vi "Update Enabled Items.vi"(10 "wheel type":string, 11 "enabled items in":T1={"Wheel Type"=TRUE, "X Position"=TRUE, "Y Position"=TRUE, "Frame Angle"=TRUE, "Wheel Name"=TRUE, "Wheel Radius"=TRUE, "Gear Ratio"=TRUE, "Forward Rotation Direction"=TRUE, "Steering Gear Ratio"=TRUE, "Motor Angle Offset"=TRUE, "Min Steering Angle"=TRUE, "Max Steering Angle"=TRUE, "Steering Range"=TRUE, "Caster Gear Ratio"=TRUE, "Forward Offset"=TRUE, "Roller Orientation"=TRUE}) -> (3 "enabled items out":T1={"Wheel Type"=TRUE, "X Position"=TRUE, "Y Position"=TRUE, "Frame Angle"=TRUE, "Wheel Name"=TRUE, "Wheel Radius"=TRUE, "Gear Ratio"=TRUE, "Forward Rotation Direction"=TRUE, "Steering Gear Ratio"=TRUE, "Motor Angle Offset"=TRUE, "Min Steering Angle"=TRUE, "Max Steering Angle"=TRUE, "Steering Range"=TRUE, "Caster Gear Ratio"=TRUE, "Forward Offset"=TRUE, "Roller Orientation"=TRUE})   [LabVIEW 2017, in "NI_Robotics_Configure Steering Frame.lvlib" / "User Defined Frame Subpanel.lvlib"]
uses:
  <vilib>/robotics/Dialog/Configure Steering Frame/User Defined Frame Subpanel/User Defined Frame Subpanel.lvlib
  <vilib>/robotics/Dialog/Configure Steering Frame/User Defined Frame Subpanel/Enabled Items.ctl
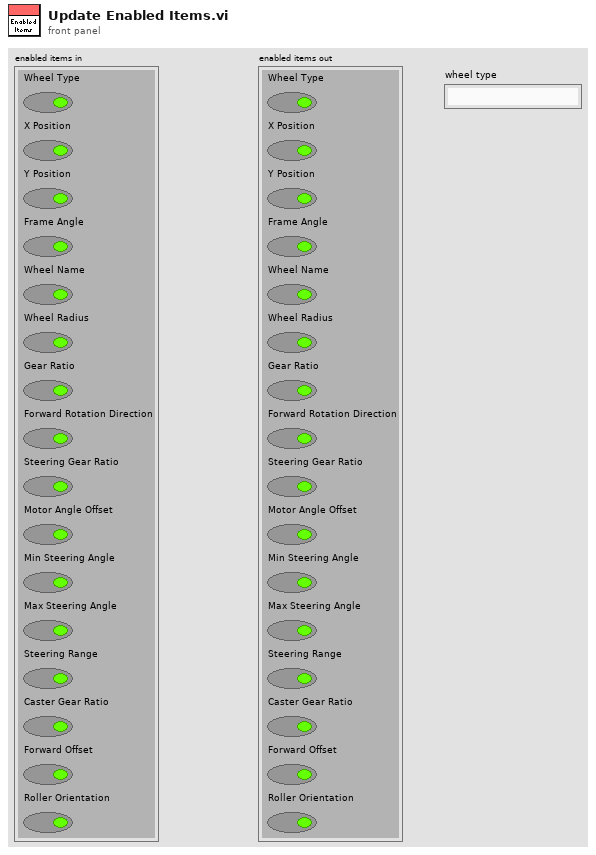
[diagram p1: front panel]
types:
  T1 = typedef "NI_Robotics_Configure Steering Frame.lvlib/User Defined Frame Subpanel.lvlib/Enabled Items.ctl" = cluster{"Wheel Type":bool, "X Position":bool, "Y Position":bool, "Frame Angle":bool, "Wheel Name":bool, "Wheel Radius":bool, "Gear Ratio":bool, "Forward Rotation Direction":bool, "Steering Gear Ratio":bool, "Motor Angle Offset":bool, "Min Steering Angle":bool, "Max Steering Angle":bool, "Steering Range":bool, "Caster Gear Ratio":bool, "Forward Offset":bool, "Roller Orientation":bool}
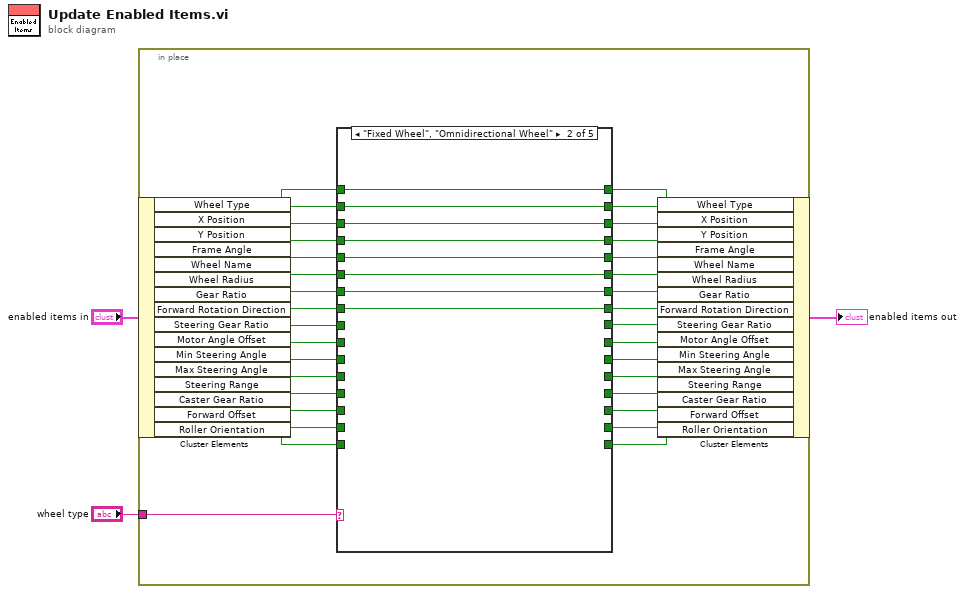
[diagram p0: block diagram]
diagram:
  n1 = in-place {
    in-place-border: "wheel type" -> [w36]
    n2 = in-place-cluster #1("enabled items in") -> ("Wheel Type"=w35:bool, "X Position"=w33:bool, "Y Position"=w31:bool, "Frame Angle"=w29:bool, "Wheel Name"=w27:bool, "Wheel Radius"=w25:bool, "Gear Ratio"=w23:bool, "Forward Rotation Direction"=w21:bool, "Steering Gear Ratio"=w19:bool, "Motor Angle Offset"=w17:bool, "Min Steering Angle"=w16:bool, "Max Steering Angle"=w15:bool, "Steering Range"=w14:bool, "Caster Gear Ratio"=w13:bool, "Forward Offset"=w12:bool, "Roller Orientation"=w11:bool)
    n3 = case shown="\"Fixed Wheel\", \"Omnidirectional Wheel\"" w36 {
      tunnel: w35 -> [w44 w52 w65 w75 w84]
      tunnel: [w44 w52 w65 w75 w84] -> w34
      tunnel: w33 -> [w43 w51 w64 w74 w83]
      tunnel: [w43 w51 w64 w74 w83] -> w32
      tunnel: w31 -> [w42 w50 w63 w73 w82]
      tunnel: [w42 w50 w63 w73 w82] -> w30
      tunnel: w29 -> [w41 w49 w62 w72 w81]
      tunnel: [w41 w49 w62 w72 w81] -> w28
      tunnel: w27 -> [w40 w48 w61 w71 w80]
      tunnel: [w40 w48 w61 w71 w80] -> w26
      tunnel: w25 -> [w39 w47 w60 w70 w79]
      tunnel: [w39 w47 w60 w70 w79] -> w24
      tunnel: w23 -> [w38 w46 w59 w69 w78]
      tunnel: [w38 w46 w59 w69 w78] -> w22
      tunnel: w21 -> [w37 w45 w57 w68 w77]
      tunnel: [w37 w45 w57 w68 w77] -> w20
      tunnel: w19 -> [_ _ w58 _ _]
      tunnel: [_ _ w58 _ _] -> w18
      tunnel: w17 -> [_ _ w56 _ _]
      tunnel: w16 -> [_ _ w55 _ _]
      tunnel: w15 -> [_ _ w54 _ _]
      tunnel: w14 -> [_ _ w53 _ _]
      tunnel: w13 -> [_ _ _ w67 _]
      tunnel: w12 -> [_ _ _ w66 _]
      tunnel: w11 -> [_ _ _ _ w76]
      tunnel: [_ _ w56 _ _] -> w10
      tunnel: [_ _ w55 _ _] -> w9
      tunnel: [_ _ w54 _ _] -> w8
      tunnel: [_ _ w53 _ _] -> w7
      tunnel: [_ _ _ w67 _] -> w6
      tunnel: [_ _ _ w66 _] -> w5
      tunnel: [_ _ _ _ w76] -> w4
      frame Default {
      }
      frame "Fixed Wheel", "Omnidirectional Wheel" {
      }
      frame "Steering Wheel" {
      }
      frame "Caster Wheel" {
      }
      frame "Mecanum Wheel" {
      }
    }
    n4 = in-place-cluster #1("Wheel Type"=w34, "X Position"=w32, "Y Position"=w30, "Frame Angle"=w28, "Wheel Name"=w26, "Wheel Radius"=w24, "Gear Ratio"=w22, "Forward Rotation Direction"=w20, "Steering Gear Ratio"=w18, "Motor Angle Offset"=w10, "Min Steering Angle"=w9, "Max Steering Angle"=w8, "Steering Range"=w7, "Caster Gear Ratio"=w6, "Forward Offset"=w5, "Roller Orientation"=w4) -> (→"enabled items out":T1)
  }
